vi "Q.Enqueue Element.vi"(4 "Data2":variant, 5 "Top of Q":bool, 6 "Data1":variant, 7 "Q Name":string, 8 "error in":errorcluster, 9 "Sub":string, 10 "Cmd":string, 11 "Q In":refnum<queue>) -> (0 "error out":errorcluster, 3 "Q Out":refnum<queue>)   [LabVIEW 2024, in "EQMF.lvlib" / "Queue Utils.lvlib"]
doc: "This VI enqueues an element to the Queue.\nIf the 'Q Name' input is not empty then it obtains the queue by name.\n If a queue is ontained by name and this queue does nto already exits, an error is generated.\nIf the 'Q Name' input is empty then it uses the 'Q In' for obtaining the queue.\n\nBy default the 'Top of Q' input is FALSE to put this element on bottom of the queue.\nSet 'Top of Q' to TRUE to enqueue this command at the top of the queue."
uses:
  Queue Utils.lvlib
  Q.Element.ctl
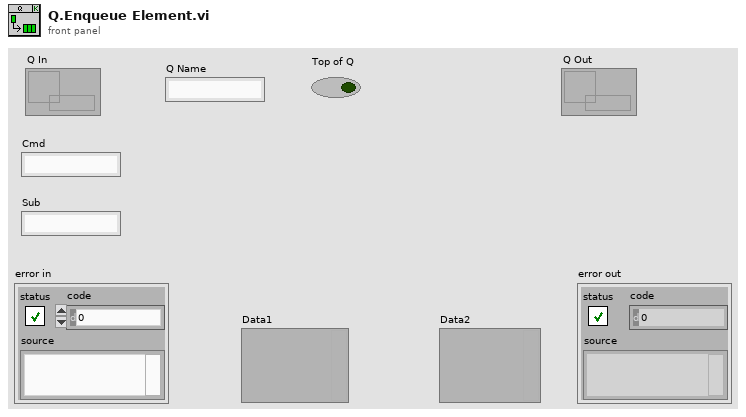
[diagram p1: front panel]
types:
  T1 = typedef "EQMF.lvlib/Queue Utils.lvlib/Q.Element.ctl" = cluster{"Cmd":string, "Sub":string, "Data1":variant, "Data2":variant}
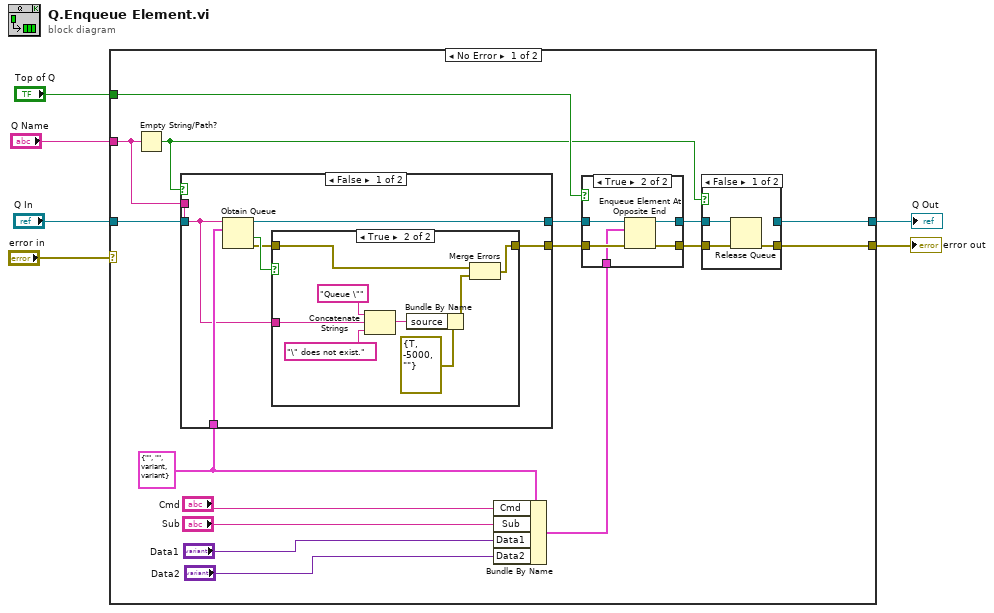
[diagram p0: block diagram]
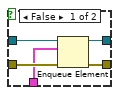
[diagram p5: hidden frame]
diagram:
  n1 = case shown="No Error" "error in" {
    selector: "error in" -> [_ w55]
    tunnel: [w15 w55] -> w6
    tunnel: "Top of Q" -> [w16 _]
    tunnel: "Q Name" -> [w11 _]
    tunnel: "Q In" -> [w12 w54]
    tunnel: [w9 w54] -> w1
    frame No Error {
      w18 = T1 {"Cmd"="", "Sub"="", "Data1"=variant, "Data2"=variant}
      n2 = Empty String/Path?(string/path=w11) -> (empty?=w10:bool)
      n3 = case shown="False" w10 {
        tunnel: [w28 _] -> w20
        tunnel: [w33 w43] -> w19
        tunnel: w11 -> [w29 _]
        tunnel: w18 -> [w32 _]
        tunnel: w12 -> [_ w43]
        frame False {
          n4 = Obtain Queue(name (unnamed)=w29, element data type=w32) -> (queue out=w33:refnum<queue>, created new?=w31:bool, error out=w30:errorcluster)  [unwired: 3 in]
          n5 = case shown="True" w31 {
            tunnel: w30 -> [w34 w36]
            tunnel: w29 -> [_ w38]
            tunnel: [w34 w35] -> w28
            frame False {
            }
            frame True {
              n6 = Concatenate Strings("Queue \"", w38, "\" does not exist.") -> (w39:string)
              n7 = Bundle By Name(cluster=errorcluster {"status"=TRUE, "code"=-5000, "source"=""} ("error constant"), "source"=w39) -> (w37:errorcluster)
              n8 = Merge Errors(w36, w37) -> (w35:errorcluster)
            }
          }
        }
        frame True {
        }
      }
      n9 = Bundle By Name(cluster=w18, "Cmd"="Cmd", "Sub"="Sub", "Data1"="Data1", "Data2"="Data2") -> (w17:T1)
      n10 = case shown="True" w16 {
        tunnel: [w46 w53] -> w14
        tunnel: [w45 w52] -> w13
        tunnel: w19 -> [w47 w51]
        tunnel: w20 -> [w48 w50]
        tunnel: w17 -> [w44 w49]
        frame False {
          n11 = Enqueue Element(queue=w47, element=w44, error in (no error)=w48) -> (queue out=w46:refnum<queue>, error out=w45:errorcluster)  [unwired: 1 in, 1 out]
        }
        frame True {
          n12 = Enqueue Element At Opposite End(queue=w51, element=w49, error in (no error)=w50) -> (queue out=w53:refnum<queue>, error out=w52:errorcluster)  [unwired: 1 in, 1 out]
        }
      }
      n13 = case shown="False" w10 {
        tunnel: [w25 w27] -> w15
        tunnel: w14 -> [w24 w26]
        tunnel: w13 -> [w23 w27]
        tunnel: [_ w26] -> w9
        frame False {
          n14 = Release Queue(queue=w24, error in (no error)=w23) -> (error out=w25:errorcluster)  [unwired: 1 in, 2 out]
        }
        frame True {
        }
      }
    }
    frame Error {
    }
  }
  "error out" <- w6
  "Q Out" <- w1
